vi "74HC153.vi"(0 "D10":bool, 1 "D11":bool, 2 "D12":bool, 3 "D13":bool, 4 "D20":bool, 5 "D21":bool, 6 "D22":bool, 7 "D23":bool, 8 "S0":bool, 9 "S1":bool, 12 "EN1":bool, 13 "EN2":bool) -> (22 "Y1":bool, 25 "Y2":bool)   [LabVIEW 2018]
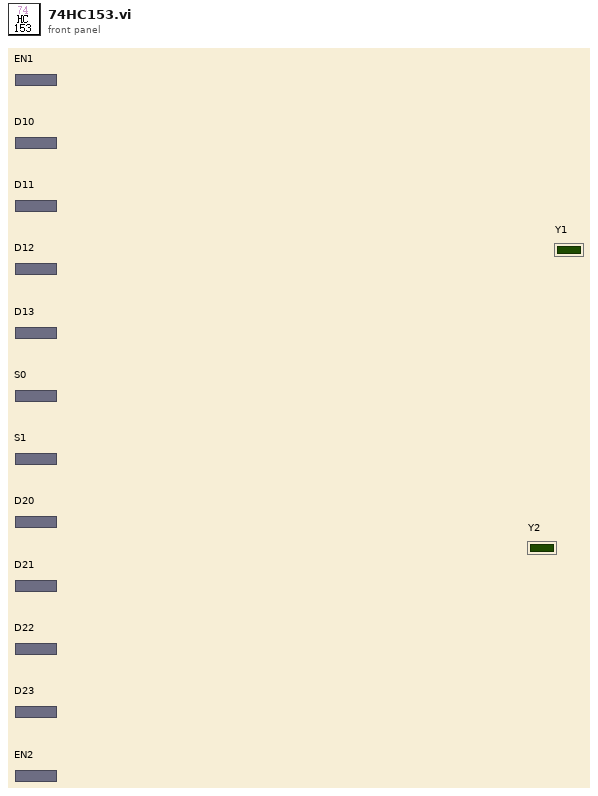
[diagram p1: front panel]
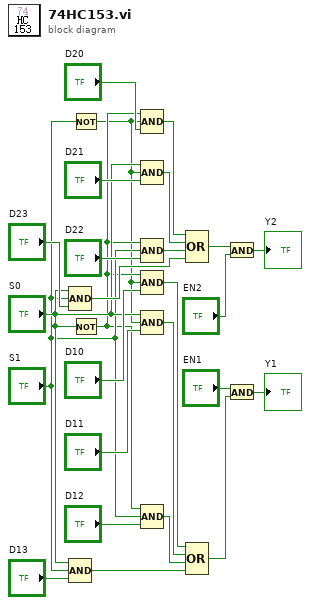
[diagram p0: block diagram]
diagram:
  n1 = Compound Arithmetic op=AND ("复合运算")("S0", "S1", "D23") -> (w12:bool)
  n2 = Compound Arithmetic op=AND ("复合运算")("S0", "S1", "D13") -> (w19:bool)
  n3 = Not(x="S1") -> (.not. x?=w1:bool)
  n4 = Not(x="S0") -> (.not. x?=w2:bool)
  n5 = Compound Arithmetic op=AND ("复合运算")(w2, w1, "D20") -> (w15:bool)
  n6 = Compound Arithmetic op=AND ("复合运算")("S0", w1, "D21") -> (w14:bool)
  n7 = Compound Arithmetic op=AND ("复合运算")(w2, "S1", "D22") -> (w13:bool)
  n8 = Compound Arithmetic op=AND ("复合运算")(w2, w1, "D10") -> (w22:bool)
  n9 = Compound Arithmetic op=AND ("复合运算")("S0", w1, "D11") -> (w21:bool)
  n10 = Compound Arithmetic op=AND ("复合运算")(w2, "S1", "D12") -> (w20:bool)
  n11 = Compound Arithmetic op=OR ("复合运算")(w15, w14, w13, w12) -> (w11:bool)
  n12 = Compound Arithmetic op=OR ("复合运算")(w22, w21, w20, w19) -> (w17:bool)
  n13 = And(x=w11, y="EN2") -> (x .and. y?=→"Y2":bool)
  n14 = And(x="EN1", y=w17) -> (x .and. y?=→"Y1":bool)
